vi "Get VI Controls.vi"(10 "DataType":string(combo)="error", 11 "VI ref.":refnum<vi>) -> (2 "#controls":i32, 3 "Controls Array":refnum<vi>[](array[refnum]))   [LabVIEW 2014]
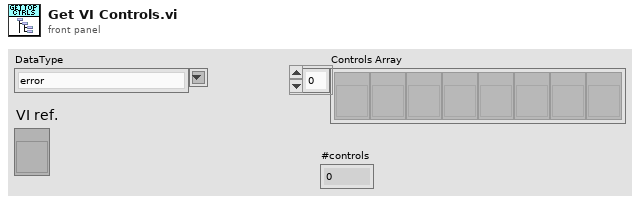
[diagram p1: front panel]
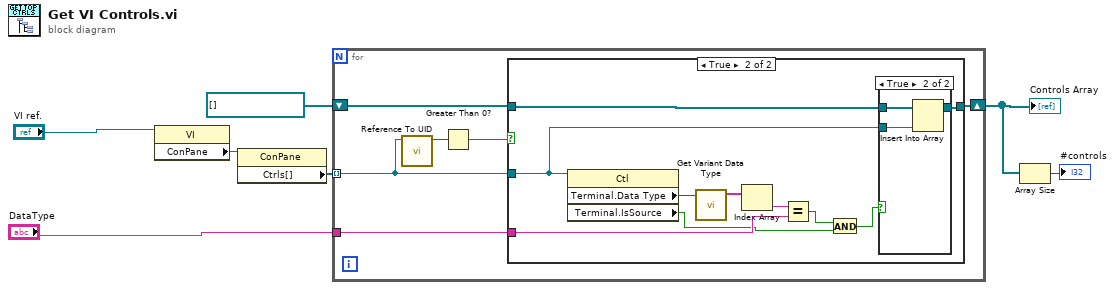
[diagram p0: block diagram]
diagram:
  n1 = property class="VI"(reference="VI ref.") -> ("ConPane"=w7:refnum<vi>)  [unwired: 1 in, 2 out]
  n2 = property class="ConPane"(reference=w7) -> ("Ctrls[]"=w6:refnum<vi>[])  [unwired: 1 in, 2 out]
  n3 = for {
    tunnel: w6 -> [w10] mode=indexing
    tunnel: "DataType" -> [w13]
    shift-right: [w11] -> w4
    shift-left: refnum<vi>[] [] -> [w12]
    n4 = call "Reference To UID.vi"("Reference"=w10) -> ("UID"=w9:i32)  [unwired: 10 in]
    n5 = Greater Than 0?(x=w9) -> (x > 0?=w8:bool)
    n6 = case shown="True" w8 {
      tunnel: w13 -> [_ w21]
      tunnel: w12 -> [w14 w20]
      tunnel: w10 -> [_ w19]
      tunnel: [w14 w18] -> w11
      frame False {
      }
      frame True {
        n7 = property class="Ctl"(reference=w19) -> ("Terminal.Data Type"=w24:variant, "Terminal.IsSource"=w15:bool)  [unwired: 1 in, 2 out]
        n8 = call "Get Variant Data Type.vi"("variant"=w24) -> ("Data Type"=w23:string[])  [unwired: 10 in]
        n9 = Index Array(array=w23) -> (element=w22:string)  [unwired: 1 in]
        n10 = Equal?(x=w22, y=w21) -> (x = y?=w17:bool)
        n11 = And(x=w17, y=w15) -> (x .and. y?=w16:bool)
        n12 = case shown="True" w16 {
          tunnel: w20 -> [w25 w28]
          tunnel: w19 -> [_ w27]
          tunnel: [w25 w26] -> w18
          frame False {
          }
          frame True {
            n13 = Insert Into Array(array=w28, new element=w27) -> (w26:refnum<vi>[])  [unwired: 1 in]
          }
        }
      }
    }
  }
  "Controls Array" <- w4
  n14 = Array Size(array=w4) -> (size(s)=→"#controls":i32)
